vi "small_rotate.vi"() -> ()   [LabVIEW 2012]
uses:
  <vilib>/NXT/Subs/LVHSConnector.ctl
  <vilib>/NXT/Subs/MotorOutput.ctl
  <vilib>/NXT/Dual Mode Library/prims/sign/sign_int.vi
  <vilib>/NXT/Dual Mode Library/Motors/MotorBrake.vi
panel:
  in  "NXT 2":T1={"Hardware"="NXT", "Flattened String"=""}
  out "degrees rotated":u16
  out "NXT":T1={"Hardware"="NXT", "Flattened String"=""}
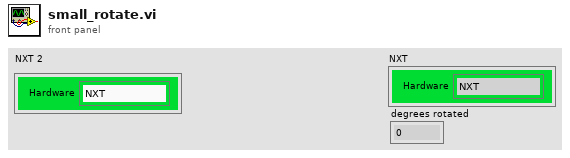
[diagram p1: front panel]
types:
  T1 = typedef "LVHSConnector.ctl" = cluster{"Hardware":string, "Flattened String":string}
  T2 = typedef "MotorOutput.ctl" = u8
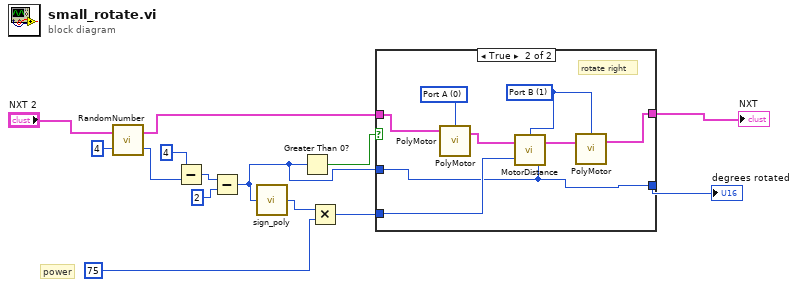
[diagram p0: block diagram]
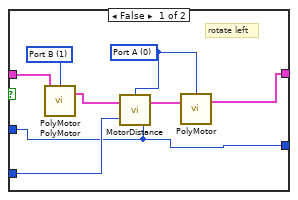
[diagram p2: hidden frame]
diagram:
  # "power"
  n1 = call <vilib>:"RandomNumber.vi"("Max Value"=u16 4, "NXT"="NXT 2") -> ("Random Number"=w9:u16, "NXT"=w14:T1)  [unwired: 1 in]
  n2 = Subtract(x=u16 4 ("Max Value"), y=w9) -> (x-y=w7:u16)
  n3 = Subtract(x=w7, y=u16 2 ("Max Value")) -> (x-y=w1:u16)
  n4 = call-poly <vilib>:"sign_poly.vi"("number"=w1) -> ("-1, 0, 1"=w5:i32)  [unwired: 4 in]
  n5 = Greater Than 0?(x=w1) -> (x > 0?=w2:bool)
  n6 = Multiply(x=w5, y=u16 75 ("Max Value")) -> (x*y=w3:i32)
  n7 = case shown="True" w2 {
    tunnel: w14 -> [w18 w26]
    tunnel: w1 -> [w15 w23]
    tunnel: w3 -> [w17 w25]
    tunnel: [w16 w24] -> w12
    tunnel: [w15 w23] -> w11
    frame False {
      w20 = T2 0 items=["Port A"=0, "Port B"=1, "Port C"=2, "Ports A & B"=4, "Ports A & C"=5, "Ports B & C"=6, "as"=3] ("Output Port (All Ports)")
      w19 = T2 1 items=["Port A"=0, "Port B"=1, "Port C"=2, "Ports A & B"=4, "Ports A & C"=5, "Ports B & C"=6, "as"=3] ("Output Port (All Ports)")
      # "rotate left"
      n8 = call-poly <vilib>:"PolyMotor.vi"("NXT"=w18) -> ()  [unwired: 3 in, 1 out]
      n9 = call-poly <vilib>:"PolyMotor.vi"("Port (All Ports)"=w19) -> ("NXT"=w22:T1)  [unwired: 3 in]
      n10 = call <vilib>:"MotorDistance.vi"("Power (75)"=w17, "Angle of Rotation (360)"=w15, "NXT"=w22, "Output Port (All Ports)"=w20) -> ("NXT"=w21:T1)
      n11 = call-poly <vilib>:"PolyMotor.vi"("NXT"=w21, "Port (All Ports)"=w20) -> ("NXT"=w16:T1)  [unwired: 2 in]
    }
    frame True {
      w28 = T2 1 items=["Port A"=0, "Port B"=1, "Port C"=2, "Ports A & B"=4, "Ports A & C"=5, "Ports B & C"=6, "as"=3] ("Output Port (All Ports)")
      w27 = T2 0 items=["Port A"=0, "Port B"=1, "Port C"=2, "Ports A & B"=4, "Ports A & C"=5, "Ports B & C"=6, "as"=3] ("Output Port (All Ports)")
      # "rotate right"
      n12 = call-poly <vilib>:"PolyMotor.vi"("NXT"=w26) -> ()  [unwired: 3 in, 1 out]
      n13 = call-poly <vilib>:"PolyMotor.vi"("Port (All Ports)"=w27) -> ("NXT"=w30:T1)  [unwired: 3 in]
      n14 = call <vilib>:"MotorDistance.vi"("Power (75)"=w25, "Angle of Rotation (360)"=w23, "NXT"=w30, "Output Port (All Ports)"=w28) -> ("NXT"=w29:T1)
      n15 = call-poly <vilib>:"PolyMotor.vi"("NXT"=w29, "Port (All Ports)"=w28) -> ("NXT"=w24:T1)  [unwired: 2 in]
    }
  }
  "NXT" <- w12
  "degrees rotated" <- w11
